vi "Init NISE Session.vi"(8 "error in (no error)":errorcluster, 11 "UI Data in":T1) -> (0 "error out":errorcluster, 3 "UI Data out":T1)   [LabVIEW 2025, in "Switch Executive Controller UI.lvlib"]
uses:
  Switch Executive Controller UI.lvlib
  UI Data.ctl
  <vilib>/SwitchExecutive/nise.llb/niSE SessionRefnum.ctl
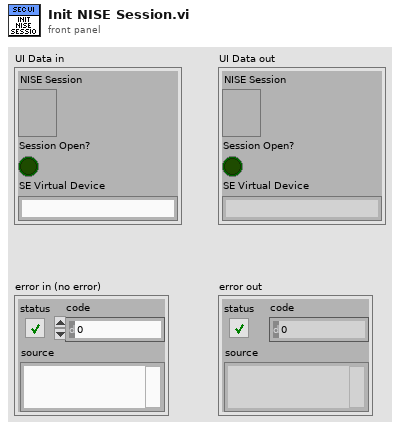
[diagram p1: front panel]
types:
  T1 = typedef "Switch Executive Controller UI.lvlib/UI Data.ctl" = cluster{"NISE Session":T2, "Session Open?":bool, "SE Virtual Device":string}
  T2 = typedef "niSE SessionRefnum.ctl" = refnum<k1>
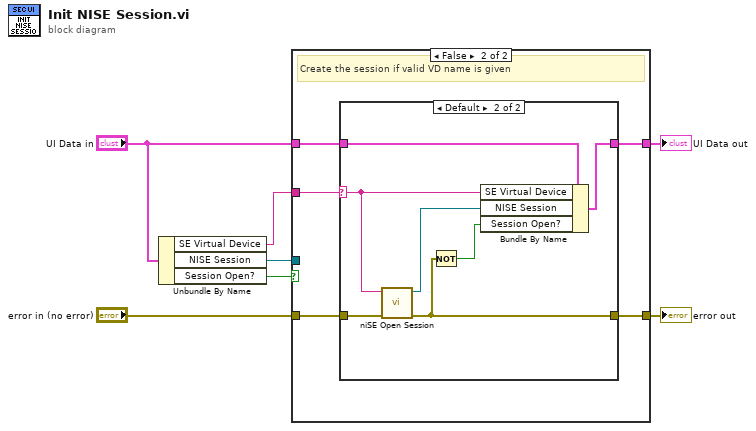
[diagram p0: block diagram]
diagram:
  n1 = Unbundle By Name("UI Data in") -> ("SE Virtual Device"=w1:string, "NISE Session"=w3:T2, "Session Open?"=w4:bool)
  n2 = case shown="False" w4 {
    tunnel: [w9 w14] -> w7
    tunnel: [w8 w13] -> w6
    tunnel: "error in (no error)" -> [w8 w12]
    tunnel: w3 -> [_ _]
    tunnel: w1 -> [_ w11]
    tunnel: "UI Data in" -> [w9 w10]
    frame True {
      # "No action if the session is already opened"
    }
    frame False {
      # "Create the session if valid VD name is given"
      n3 = case shown="Default" w11 {
        selector: w11 -> [_ w20]
        tunnel: w12 -> [w16 w23]
        tunnel: [w16 w18] -> w13
        tunnel: w10 -> [w15 w22]
        tunnel: [w15 w19] -> w14
        frame "" {
        }
        frame Default {
          n4 = call <vilib>:"niSE Open Session.vi"("error in (no error)"=w23, "Virtual Device Name (SwitchConfiguration1)"=w20) -> ("error out"=w18:errorcluster, "NISE Session (out)"=w21:T2)  [unwired: 4 in]
          n5 = Not(x=w18) -> (.not. x?=w17:bool)
          n6 = Bundle By Name(cluster=w22, "SE Virtual Device"=w20, "NISE Session"=w21, "Session Open?"=w17) -> (w19:T1)
        }
      }
    }
  }
  "UI Data out" <- w7
  "error out" <- w6
